vi "Result by Index.vi"(7 "Mark Visited? (F)":bool, 8 "error in (no error)":errorcluster, 10 "Result Index":i32, 11 "Search in":refnum<class "Search.lvclass">) -> (0 "error out":errorcluster, 2 "Result":refnum<class "Search Result.lvclass">, 3 "Search out":refnum<class "Search.lvclass">)   [LabVIEW 2016, in "Better Search.lvlib" / "Search.lvclass"]
uses:
  Search.lvclass
  Search Result/Search Result.lvclass
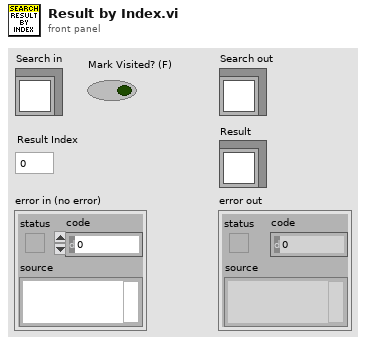
[diagram p1: front panel]
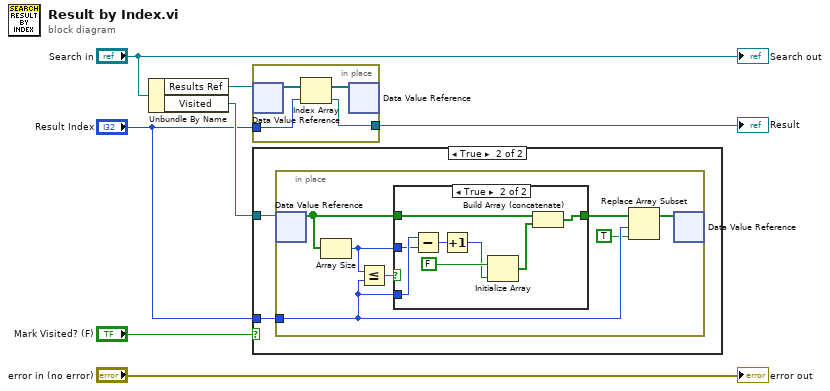
[diagram p0: block diagram]
diagram:
  n1 = Unbundle By Name("Search in") -> ("Results Ref"=w6:refnum<data-value>, "Visited"=w3:refnum<data-value>)
  n2 = in-place {
    in-place-border: "Result Index" -> [w9]
    in-place-border: [w8] -> w4
    n3 = in-place-dvr #1(w6) -> (w10:refnum<class "Search Result.lvclass">[])  [unwired: 1 out]
    n4 = Index Array(array=w10, index=w9) -> (element=w8:refnum<class "Search Result.lvclass">)
    n5 = in-place-dvr #1(w10) -> ()  [unwired: 2 out]
  }
  "Result" <- w4
  n6 = case shown="True" "Mark Visited? (F)" {
    tunnel: w3 -> [_ w12]
    tunnel: "Result Index" -> [_ w11]
    frame False {
    }
    frame True {
      n7 = in-place {
        in-place-border: w11 -> [w14]
        n8 = in-place-dvr #2(w12) -> (w17:bool[])  [unwired: 1 out]
        n9 = Array Size(array=w17) -> (size(s)=w19:i32)
        n10 = Less Or Equal?(x=w19, y=w14) -> (x <= y?=w18:bool)
        n11 = case shown="True" w18 {
          tunnel: w19 -> [_ w27]
          tunnel: w14 -> [_ w28]
          tunnel: w17 -> [w20 w24]
          tunnel: [w20 w22] -> w16
          frame False {
          }
          frame True {
            n12 = Subtract(x=w28, y=w27) -> (x-y=w26:i32)
            n13 = Increment(x=w26) -> (x+1=w21:i32)
            n14 = Initialize Array(FALSE, w21) -> (w23:bool[])
            n15 = Build Array (concatenate)(w24, w23) -> (w22:bool[])
          }
        }
        n16 = Replace Array Subset(array=w16, new element=TRUE ("new element/subarray"), index=w14) -> (w15:bool[])
        n17 = in-place-dvr #2(w15) -> ()  [unwired: 2 out]
      }
    }
  }
  "error out" <- "error in (no error)"
  "Search out" <- "Search in"
